vi "regression_matrix.vi"(3 "W_prev":dbl[](array[numeric]), 4 "EW":cluster{"E":dbl[], "W":dbl[]}, 5 "desired":cluster{"Ed":dbl[], "Wd":dbl[], "Wd_dot":dbl[]}, 6 "m":dbl) -> (0 "W_Prev":dbl[](array[numeric])=[0.4, 0.1, -0.4], 1 "Y_icl_sys":dbl[][](array[numeric]), 2 "Y_sys":dbl[][](array[numeric]))   [LabVIEW 2018]
uses:
  <vilib>/imath/engines/lvmath2/RunTimeEngine/BuiltInFunctions/reshapemx/NIMS_[GV]_reshapemx.vi
  <instcachedir>/0/NIMS_[GV]_reshapemx_FC3E9BFA29934BE8A99DD7B75AE8F89C.lvgen/NIMS_[GV]_reshapemx_FC3E9BFA29934BE8A99DD7B75AE8F89C_000.vi
  <vilib>/imathl/engines/lvmath/Functions/Error Handling/Create Error.vi
  <vilib>/imath/engines/lvmath2/RunTimeEngine/IndexRead/NIMS V(S).vi
  <instcachedir>/0/NIMS V(S)_0488751826AF41519A22953C041130DC.lvgen/NIMS V(S)_0488751826AF41519A22953C041130DC_000.vi
  <vilib>/imath/engines/lvmath2/RunTimeEngine/ErrorHandling/NIMS_Create Error From Enums.vi
  <vilib>/imath/engines/lvmath2/RunTimeEngine/ArithmeticOperatorToken/NIMS_ArithmeticOperator_minus.vi
  <instcachedir>/0/NIMS_ArithmeticOperator_minus_C4D0373119CC411691B2E50DF2E09F22.lvgen/NIMS_ArithmeticOperator_minus_C4D0373119CC411691B2E50DF2E09F22_003.vi
  <vilib>/imath/engines/lvmath2/RunTimeEngine/NodeEndStatement/NIMS_NodeEndStatement_Output.vi
  <instcachedir>/0/NIMS_NodeEndStatement_Output_53EC0D466D134D7ABD903AC30B43404B.lvgen/NIMS_NodeEndStatement_Output_53EC0D466D134D7ABD903AC30B43404B_002.vi
  <vilib>/imath/engines/lvmath2/RunTimeEngine/ErrorHandling/NIMS_Finalize Error.vi
  <vilib>/imath/engines/lvmath2/RunTimeEngine/ArithmeticOperatorToken/NIMS_ArithmeticOperator_multmx(M,CV)-internal.vi
  <instcachedir>/0/NIMS_ArithmeticOperator_multmx(M,CV)-internal_5287250D8D1D4A3E9F77F5DF08D432E0.lvgen/NIMS_ArithmeticOperator_multmx(M,CV)-internal_5287250D8D1D4A3E9F77F5DF08D432E0_001.vi
  <vilib>/imath/engines/lvmath2/RunTimeEngine/ArithmeticOperatorToken/NIMS_ArithmeticOperator_multmx.vi
  <instcachedir>/0/NIMS_ArithmeticOperator_multmx_622CA76F9646436AB036D42A9A1CE0E6.lvgen/NIMS_ArithmeticOperator_multmx_622CA76F9646436AB036D42A9A1CE0E6_004.vi
  <vilib>/imath/engines/lvmath2/RunTimeEngine/ArithmeticOperatorToken/NIMS_ArithmeticOperator_multmx(M,CV).vi
  <instcachedir>/0/NIMS_ArithmeticOperator_multmx(M,CV)_2F1CD6A2FE4F4213A4AD1C901C2750F5.lvgen/NIMS_ArithmeticOperator_multmx(M,CV)_2F1CD6A2FE4F4213A4AD1C901C2750F5_000.vi
  <instcachedir>/0/NIMS_ArithmeticOperator_minus_C4D0373119CC411691B2E50DF2E09F22.lvgen/NIMS_ArithmeticOperator_minus_C4D0373119CC411691B2E50DF2E09F22_002.vi
  <vilib>/imath/engines/lvmath2/RunTimeEngine/IndexRead/NIMS M(S).vi
  <instcachedir>/0/NIMS M(S)_B826C018497E4940AE96BD27B540B6FB.lvgen/NIMS M(S)_B826C018497E4940AE96BD27B540B6FB_000.vi
  <vilib>/imath/engines/lvmath2/RunTimeEngine/RowToken/NIMS_RowToken_M_M.vi
  <instcachedir>/0/NIMS_RowToken_M_M_9381229BAB584C0281F245468A1A9A6C.lvgen/NIMS_RowToken_M_M_9381229BAB584C0281F245468A1A9A6C_004.vi
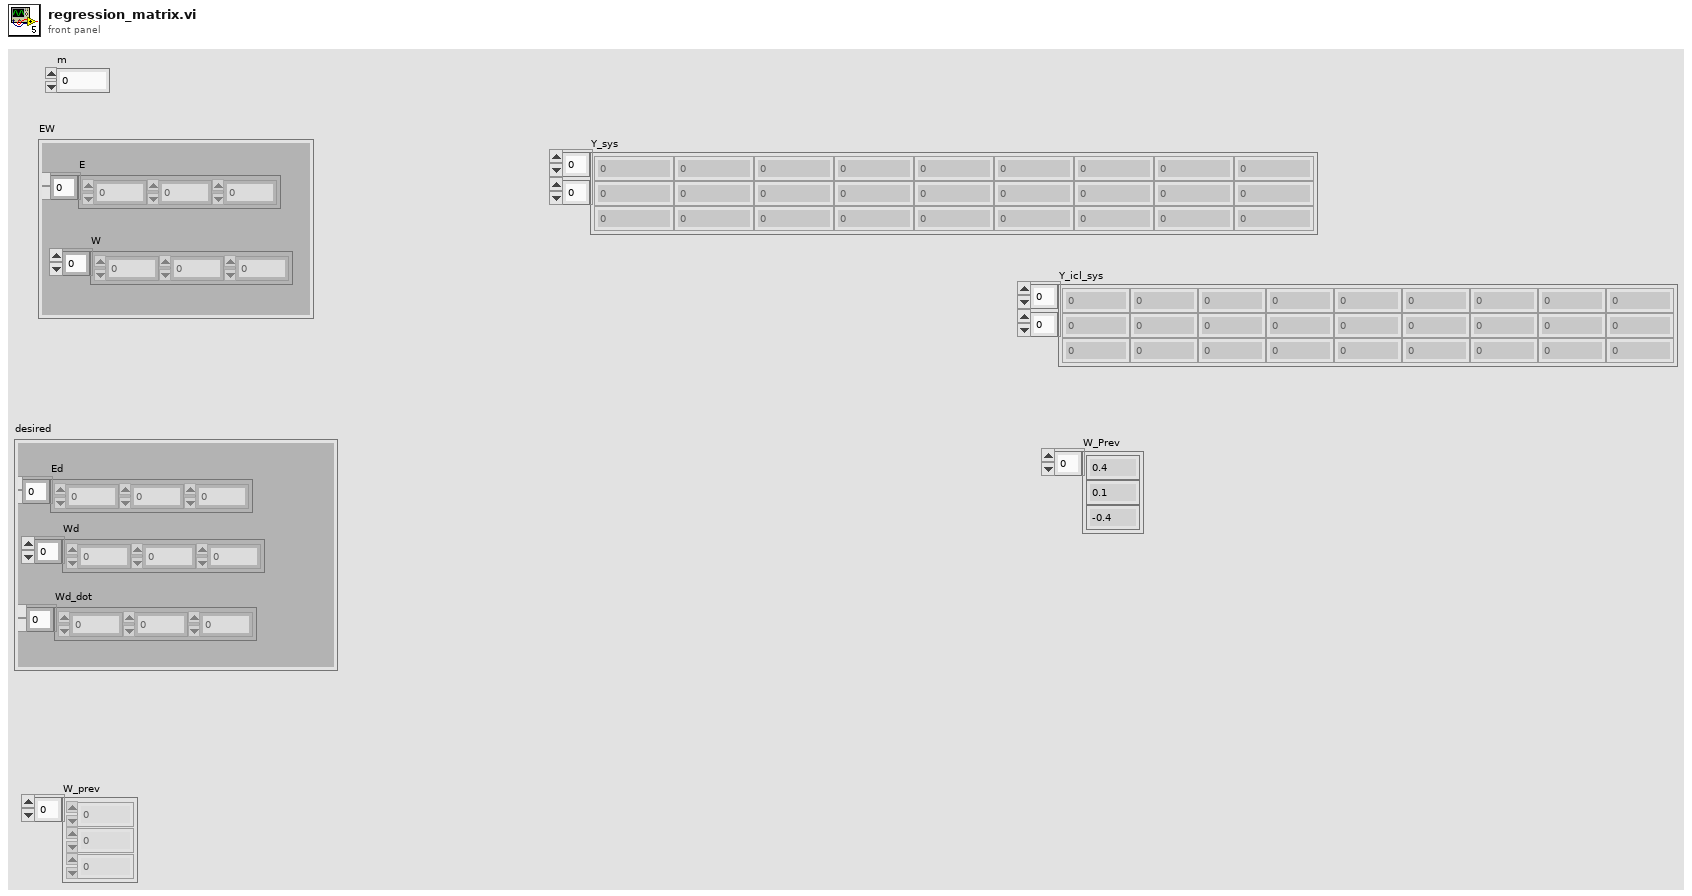
[diagram p1: front panel]
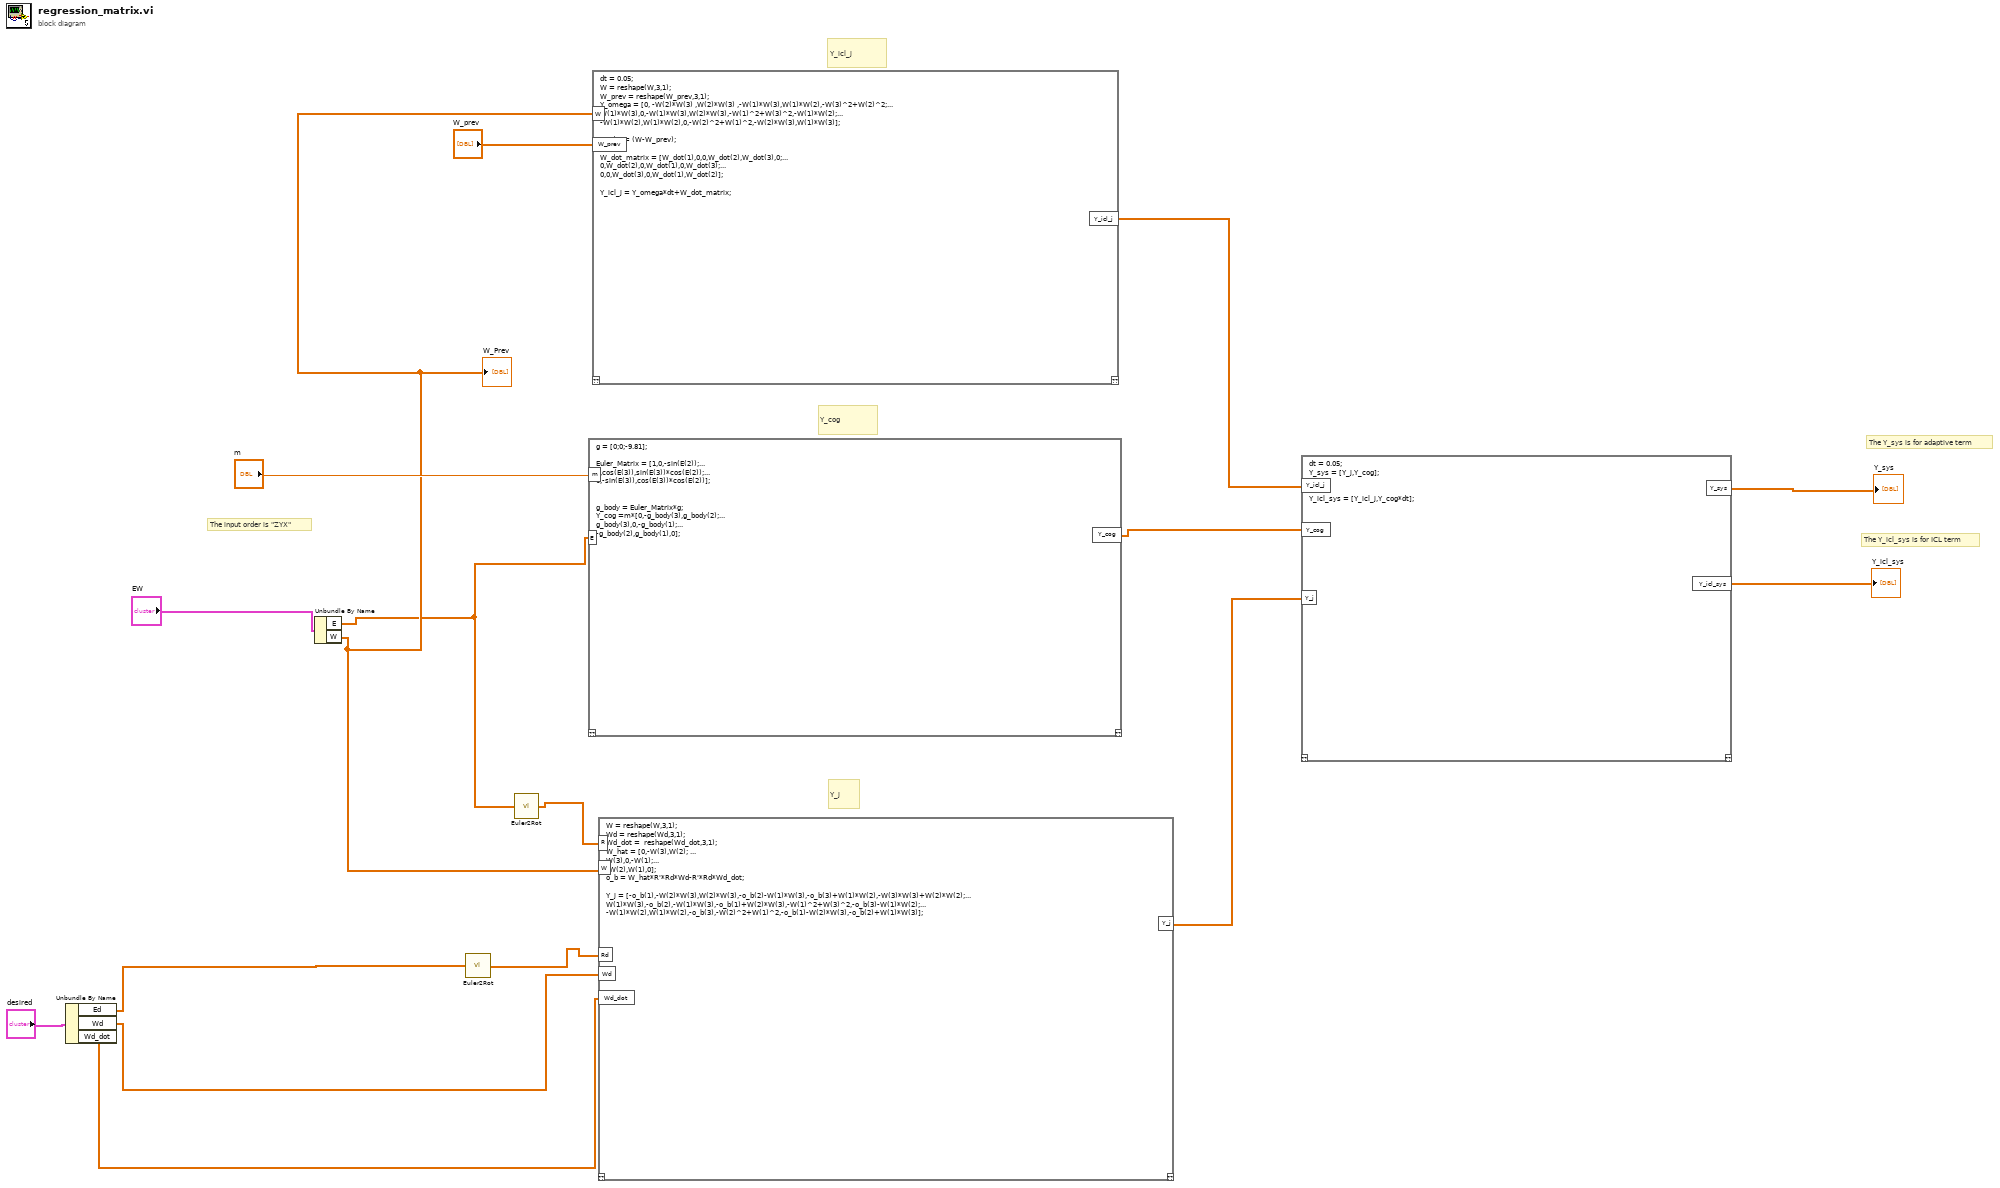
[diagram p0: block diagram]
diagram:
  # "The input order is \"ZYX\""
  # "The Y_icl_sys is for ICL term"
  # "The Y_sys is for adaptive term"
  # "Y_j"
  # "Y_icl_j"
  # "Y_cog"
  n1 = Unbundle By Name("desired") -> ("Ed"=w3:dbl[], "Wd"=w6:dbl[], "Wd_dot"=w5:dbl[])
  n2 = Unbundle By Name("EW") -> ("E"=w1:dbl[], "W"=w8:dbl[])
  "W_Prev" <- w8
  n3 = call "Euler2Rot.vi"("Ed"=w3) -> ("Rd"=w4:dbl[][])
  n4 = call "Euler2Rot.vi"("Ed"=w1) -> ("Rd"=w2:dbl[][])
  n5 = mathscript code="g = [0;0;-9.81];\n\nEuler_Matrix = [1,0,-sin(E(2));...\n0,cos(E(3)),sin(E(3))*cos(E(2));...\n0,-sin(E(3)),cos(E(3))*cos(E(2))];\n\n\ng_body = Euler_Matrix*g;\nY_cog =m*[0,-g_body(3),g_body(2);...\ng_body(3),0,-g_body(1);...\n-g_body(2),g_body(1),0];"("m"="m", "E"=w1) -> ("Y_cog"=w15:dbl[][])  [unwired: 1 in, 1 out]
  n6 = mathscript code="dt = 0.05;\nW = reshape(W,3,1);\nW_prev = reshape(W_prev,3,1);\nY_omega = [0, -W(2)*W(3) ,W(2)*W(3) ,-W(1)*W(3),W(1)*W(2),-W(3)^2+W(2)^2;...\nW(1)*W(3),0,-W(1)*W(3),W(2)*W(3),-W(1)^2+W(3)^2,-W(1)*W(2);...\n-W(1)*W(2),W(1)*W(2),0,-W(2)^2+W(1)^2,-W(2)*W(3),W(1)*W(3)];\n\nW_dot = (W-W_prev);\n\nW_dot_matrix = [W_dot(1),0,0,W_dot(2),W_dot(3),0;...\n0,W_dot(2),0,W_dot(1),0,W_dot(3);...\n0,0,W_dot(3),0,W_dot(1),W_dot(2)];\n\nY_icl_j = Y_omega*dt+W_dot_matrix;"("W"=w8, "W_prev"="W_prev") -> ("Y_icl_j"=w16:dbl[][])  [unwired: 1 in, 1 out]
  n7 = mathscript code="W = reshape(W,3,1);\nWd = reshape(Wd,3,1);\nWd_dot =  reshape(Wd_dot,3,1);\nW_hat = [0,-W(3),W(2); ...\nW(3),0,-W(1);...\n-W(2),W(1),0];\no_b = W_hat*R'*Rd*Wd-R'*Rd*Wd_dot;\n\nY_j = [-o_b(1),-W(2)*W(3),W(2)*W(3),-o_b(2)-W(1)*W(3),-o_b(3)+W(1)*W(2),-W(3)*W(3)+W(2)*W(2);...\nW(1)*W(3),-o_b(2),-W(1)*W(3),-o_b(1)+W(2)*W(3),-W(1)^2+W(3)^2,-o_b(3)-W(1)*W(2);...\n-W(1)*W(2),W(1)*W(2),-o_b(3),-W(2)^2+W(1)^2,-o_b(1)-W(2)*W(3),-o_b(2)+W(1)*W(3)];"("W"=w8, "Rd"=w4, "R"=w2, "Wd_dot"=w5, "Wd"=w6) -> ("Y_j"=w14:dbl[][])  [unwired: 1 in, 1 out]
  n8 = mathscript code="dt = 0.05;\nY_sys = [Y_j,Y_cog];\n\n\nY_icl_sys = [Y_icl_j,Y_cog*dt];"("Y_icl_j"=w16, "Y_cog"=w15, "Y_j"=w14) -> ("Y_sys"=→"Y_sys":dbl[][], "Y_icl_sys"=→"Y_icl_sys":dbl[][])  [unwired: 1 in, 1 out]
